vi "Drive away from attack.vi"(5 "max reverse velocity (m/s)":dbl, 7 "max angular velocity (rad/s)":dbl=1.0, 8 "error in (no error)":errorcluster, 9 "dir1":dbl, 10 "find":bool, 11 "angle":dbl) -> (0 "error out":errorcluster, 2 "steering frame velocity":dbl[](array[numeric]))   [LabVIEW 2012]
doc: "Sets the steering frame velocity so that the robot moves in reverse and rotates towards the gap."
uses:
  <vilib>/imath/engines/lvmath2/RunTimeEngine/ErrorHandling/NIMS_Finalize Error.vi
  <vilib>/imath/engines/lvmath2/RunTimeEngine/BuiltInFunctions/abs/NIMS_abs(signed).vi
  <instcachedir>/0/NIMS_abs(signed)_C4FCB8E6058B49B797C7C8D53CA5F6EC.lvgen/NIMS_abs(signed)_C4FCB8E6058B49B797C7C8D53CA5F6EC_000.vi
  <vilib>/imath/engines/lvmath2/RunTimeEngine/VariableToken/NIMS_VariableToken_CondDefined.vi
  <instcachedir>/0/NIMS_VariableToken_CondDefined_295AAB8C64C949DA8EA45AB7820AF759.lvgen/NIMS_VariableToken_CondDefined_295AAB8C64C949DA8EA45AB7820AF759_003.vi
  <vilib>/imathl/engines/lvmath/Functions/Error Handling/Create Error.vi
  <instcachedir>/0/NIMS_VariableToken_CondDefined_295AAB8C64C949DA8EA45AB7820AF759.lvgen/NIMS_VariableToken_CondDefined_295AAB8C64C949DA8EA45AB7820AF759_004.vi
  <vilib>/imath/engines/lvmath/Functions/Error Handling/MergeErrorsWrapper.vi
  <vilib>/imath/engines/lvmath2/RunTimeEngine/NodeEndStatement/NIMS_NodeEndStatement_Output.vi
  <instcachedir>/0/NIMS_NodeEndStatement_Output_53EC0D466D134D7ABD903AC30B43404B.lvgen/NIMS_NodeEndStatement_Output_53EC0D466D134D7ABD903AC30B43404B_013.vi
  <instcachedir>/0/NIMS_NodeEndStatement_Output_53EC0D466D134D7ABD903AC30B43404B.lvgen/NIMS_NodeEndStatement_Output_53EC0D466D134D7ABD903AC30B43404B_001.vi
  <instcachedir>/0/NIMS_NodeEndStatement_Output_53EC0D466D134D7ABD903AC30B43404B.lvgen/NIMS_NodeEndStatement_Output_53EC0D466D134D7ABD903AC30B43404B_012.vi
panel:
  out "t":u32
  out "angle 2":dbl
  in  "kaiguan":bool
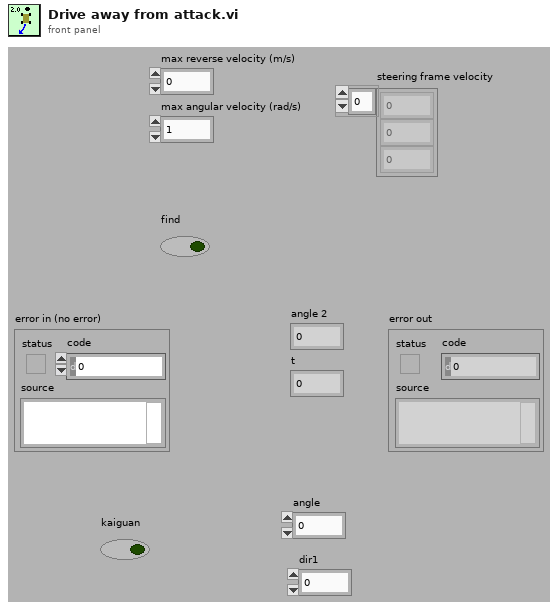
[diagram p1: front panel]
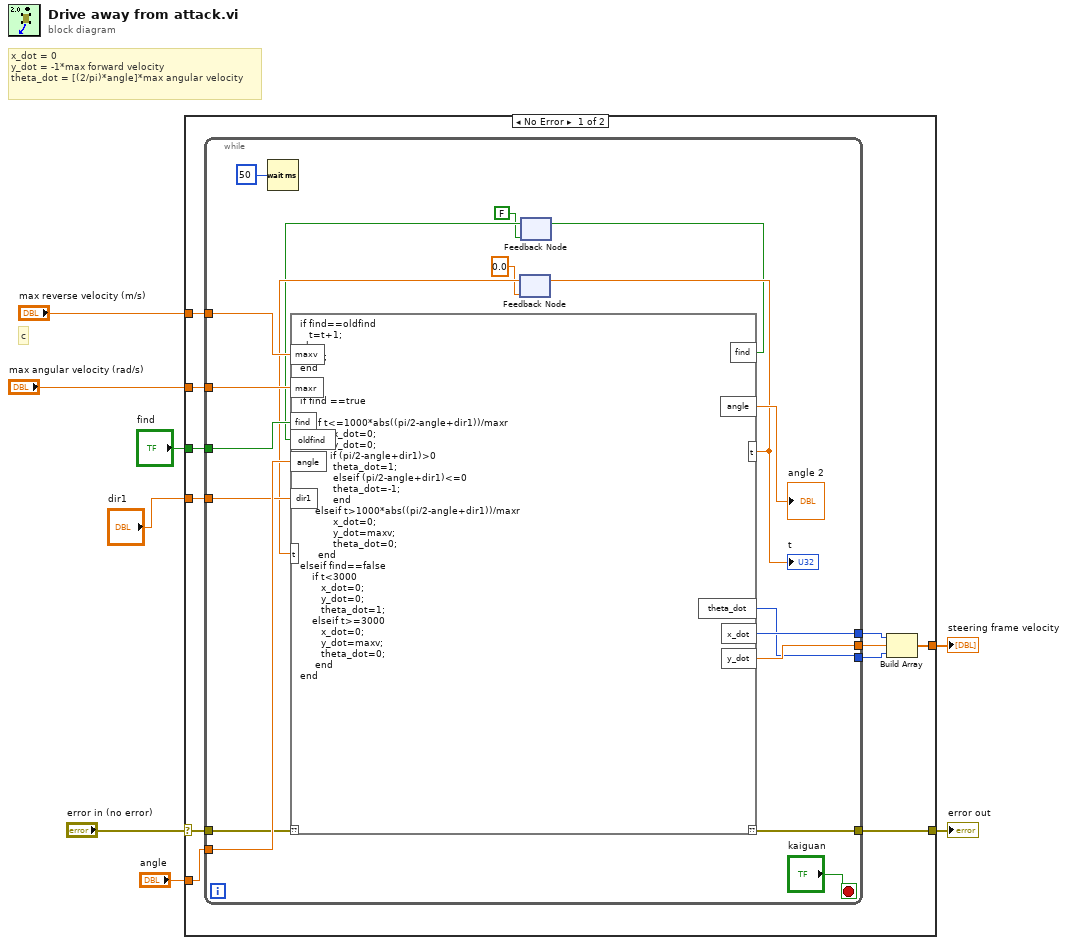
[diagram p0: block diagram]
diagram:
  # "c"
  # "x_dot = 0\ny_dot = -1*max forward velocity\ntheta_dot = [(2/pi)*angle]*max angular velocity"
  n1 = case shown="No Error" "error in (no error)" {
    selector: "error in (no error)" -> [w13 w373]
    tunnel: [w12 w373] -> w7
    tunnel: "max reverse velocity (m/s)" -> [w18 _]
    tunnel: "max angular velocity (rad/s)" -> [w17 _]
    tunnel: [w19 _] -> w2
    tunnel: "find" -> [w16 _]
    tunnel: "dir1" -> [w14 _]
    tunnel: "angle" -> [w15 _]
    frame No Error {
      n2 = while {
        tunnel: w18 -> [w34]
        tunnel: w17 -> [w33]
        tunnel: w16 -> [w29]
        tunnel: w15 -> [w38]
        tunnel: w14 -> [w37]
        tunnel: w13 -> [w36]
        tunnel: [w35] -> w12
        tunnel: [w32] -> w11
        tunnel: [w31] -> w10
        tunnel: [w30] -> w9
        stop <- "kaiguan" stop-if-true
        n3 = Wait (ms)(milliseconds to wait=u32 50) -> ()  [unwired: 1 out]
        n4 = feedback #1(0.0 ("t")) -> (w24:dbl)
        n5 = feedback #2(FALSE ("find")) -> (w22:bool)
        n6 = mathscript code="if find==oldfind\n   t=t+1;\nelse\n  t=0;\nend\n\n\nif find ==true\n     \n     if t<=1000*abs((pi/2-angle+dir1))/maxr\n           x_dot=0;\n           y_dot=0; \n          if (pi/2-angle+dir1)>0\n           theta_dot=1;\n           elseif (pi/2-angle+dir1)<=0\n           theta_dot=-1;\n           end\n     elseif t>1000*abs((pi/2-angle+dir1))/maxr\n           x_dot=0;\n           y_dot=maxv;\n           theta_dot=0;\n      end\nelseif find==false\n    if t<3000\n       x_dot=0;\n       y_dot=0;\n       theta_dot=1;\n    elseif t>=3000\n       x_dot=0;\n       y_dot=maxv;\n       theta_dot=0;\n     end\nend"("??"=w36, "maxv"=w34, "maxr"=w33, "find"=w29, "angle"=w38, "dir1"=w37, "t"=w24, "oldfind"=w22) -> ("??"=w35:errorcluster, "theta_dot"=w30:i32, "x_dot"=w32:i32, "y_dot"=w31:dbl, "t"=w25:dbl, "angle"=→"angle 2":dbl, "find"=w23:bool)
        "t" <- w25
        n7 = feedback-in #1(w25) -> ()
        n8 = feedback-in #2(w23) -> ()
      }
      n9 = Build Array(w11, w10, w9) -> (w19:dbl[])
    }
    frame Error {
    }
  }
  "error out" <- w7
  "steering frame velocity" <- w2
